vi "LatestAPLPath.vi"(8 "Error In":errorcluster, 9 "APL Search String":T1(ring), 11 "Folder Path":path=path "\\\\itnas.appl.ge.com\\technology/Electronics/InProcess/Software/ci_builds/2015_VA_Washer") -> (0 "Error Out":errorcluster, 1 "Report text":string, 2 "Found ?":bool, 3 "File Path":path=path "\\\\itnas.appl.ge.com\\technology/Electronics/InProcess/Software/ci_builds/2015_VA_Washer/2015-03-06_03-42-38(Build-1952)/Binaries/2015VAWasher_Param_QA_Cycle_1_62_99_1.apl")   [LabVIEW 2016, in "TL27.lvlib"]
doc: "This VI will search for the most recent version of software apls and return its path. You can search for various firware or xml apls.\n\nIf not found it will return an empty path, as well and boolean and report text."
uses:
  Projects/TL27.lvlib
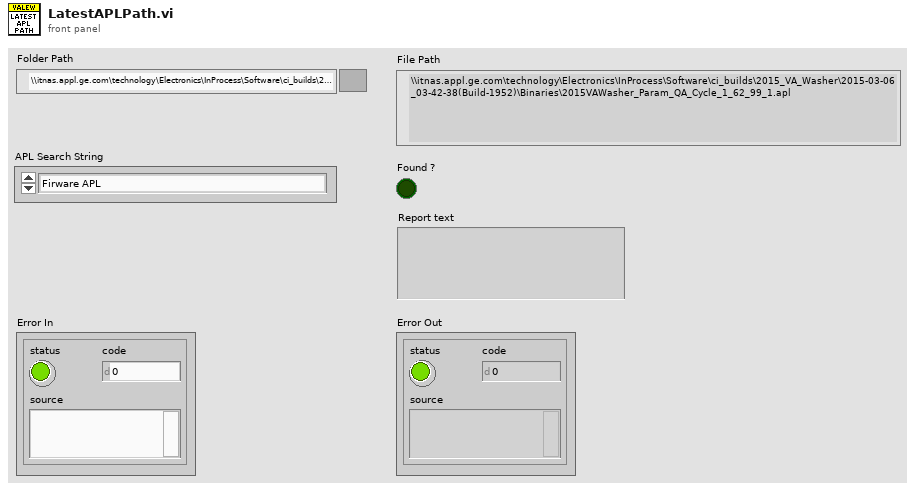
[diagram p1: front panel]
types:
  T1 = enum16{"Firware APL", "QA XML APL", "System XML", "QA Cycle XML APL", "Reliability Cycle XML", "ElectronicsCycles", "ERD Definitions XML"}
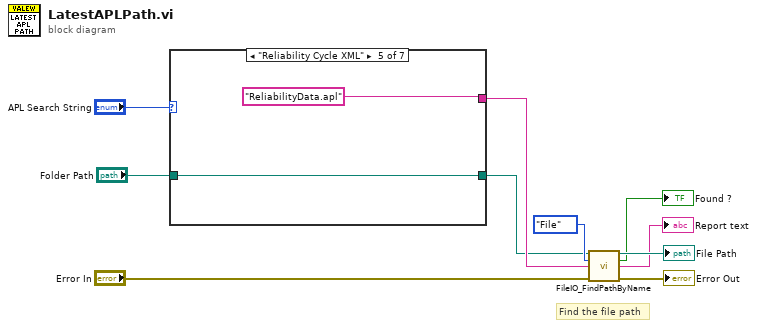
[diagram p0: block diagram]
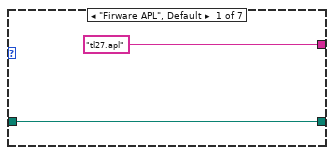
[diagram p2: hidden frame]
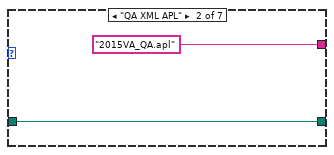
[diagram p3: hidden frame]
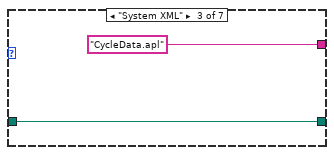
[diagram p4: hidden frame]
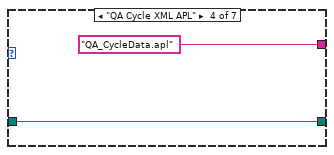
[diagram p5: hidden frame]
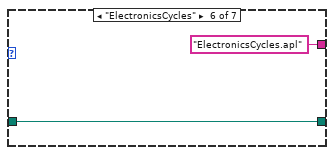
[diagram p6: hidden frame]
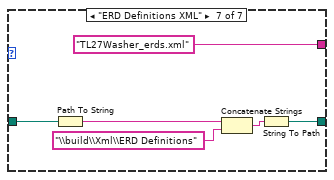
[diagram p7: hidden frame]
diagram:
  # "Find the file path"
  n1 = case shown="\"Reliability Cycle XML\"" "APL Search String" {
    tunnel: ["tl27.apl" "2015VA_QA.apl" "CycleData.apl" "QA_CycleData.apl" "ReliabilityData.apl" "ElectronicsCycles.apl" "TL27Washer_erds.xml"] -> w7
    tunnel: [w11 w13 w15 w17 w19 w21 w23] -> w1
    tunnel: "Folder Path" -> [w11 w13 w15 w17 w19 w21 w24]
    frame "Firware APL", Default {
    }
    frame "QA XML APL" {
    }
    frame "System XML" {
    }
    frame "QA Cycle XML APL" {
    }
    frame "Reliability Cycle XML" {
    }
    frame "ElectronicsCycles" {
    }
    frame "ERD Definitions XML" {
      n2 = Path To String(path=w24) -> (string=w28:string)
      n3 = Concatenate Strings(w28, "\\build\\Xml\\ERD Definitions" ("string")) -> (w26:string)
      n4 = String To Path(string=w26) -> (path=w23:path)
    }
  }
  n5 = call "FileIO_FindPathByName.vi"("Path In"=w1, "File or Folder ?"=enum16{"Folder", "File"}."File", "File/Folder Search String"=w7, "Error In"="Error In") -> ("Path Out"=→"File Path":path, "Found ?"=→"Found ?":bool, "Report Text"=→"Report text":string, "Error Out"=→"Error Out":errorcluster)  [unwired: 8 in]
